vi "dbTest.vi"() -> ()   [LabVIEW 2015]
uses:
  C:/Users/Arkadiusz/SkyDrive/Dokumenty/Visual Studio 2015/Projects/NordicDatabaseDLL/NordicDatabaseDLL/bin/Debug/NordicDatabaseDLL.dll
  SkyDrive/Dokumenty/Visual Studio 2015/Projects/NordicDatabaseDLL/NordicDatabaseDLL/bin/Debug/NordicDatabaseDLL.dll
panel:
  in  "Boolean":bool
  in  "stop":bool
  in  "temperatureData":sgl[](array[numeric])
  out "SelectDataTemperature":sgl[](array[numeric])
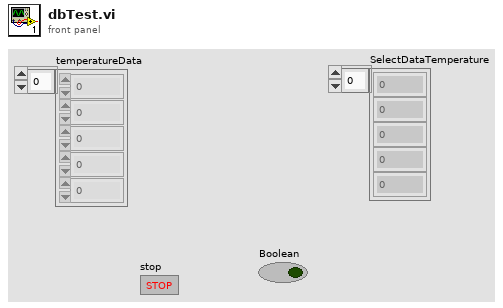
[diagram p1: front panel]
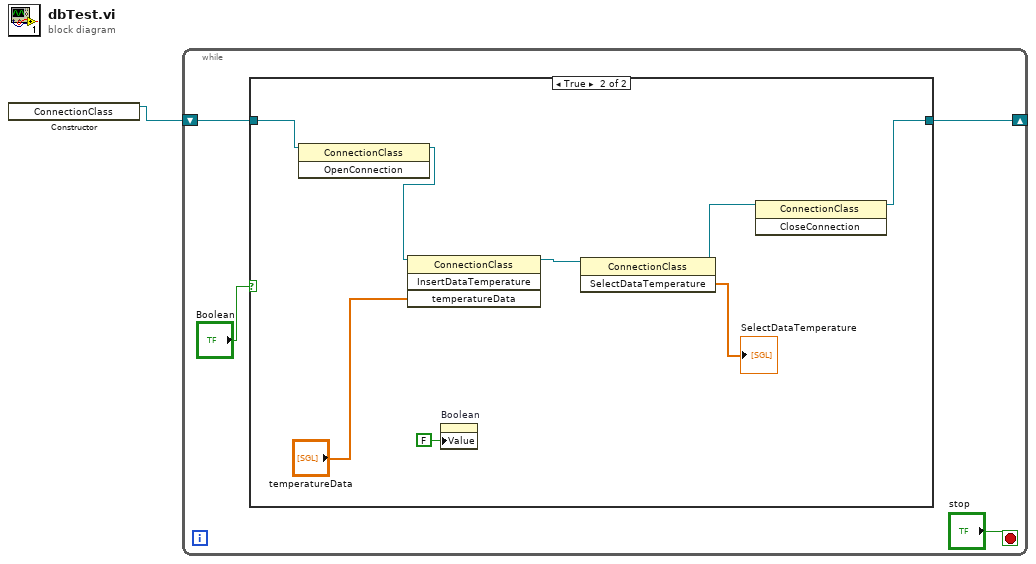
[diagram p0: block diagram]
diagram:
  n1 = constructor class="ConnectionClass"() -> (reference out=w1:refnum<k24>)  [unwired: 3 in, 2 out]
  n2 = while {
    shift-right: [w2] -> _
    shift-left: w1 -> [w5]
    stop <- "stop" stop-if-true
    n3 = case shown="True" "Boolean" {
      tunnel: w5 -> [w6 w9]
      tunnel: [w6 w10] -> w2
      frame False {
      }
      frame True {
        n4 = invoke class="ConnectionClass" method="OpenConnection"(reference=w9) -> (reference out=w8:refnum<k24>)  [unwired: 2 in, 2 out]
        n5 = invoke class="ConnectionClass" method="InsertDataTemperature"(reference=w8, "temperatureData"="temperatureData") -> (reference out=w13:refnum<k24>)  [unwired: 2 in, 3 out]
        n6 = property on="Boolean" class="Bool (strict)"("Value"=FALSE ("Boolean")) -> ()  [unwired: 2 in, 2 out]
        n7 = invoke class="ConnectionClass" method="SelectDataTemperature"(reference=w13) -> (reference out=w12:refnum<k24>, "SelectDataTemperature"=→"SelectDataTemperature":sgl[])  [unwired: 2 in, 1 out]
        n8 = invoke class="ConnectionClass" method="CloseConnection"(reference=w12) -> (reference out=w10:refnum<k24>)  [unwired: 2 in, 2 out]
      }
    }
  }
